vi "Values.vi"(11 "Result Row in":refnum<class "Result Row.lvclass">) -> (2 "Value":refnum<class "Type.lvclass">[](array[class]))   [LabVIEW 2022 SP3, in "Conditum.lvlib" / "Result Row.lvclass"]
uses:
  Result Row.lvclass
  Result Row.lvclass/Result Row.ctl
  Columns/Type/Type.lvclass
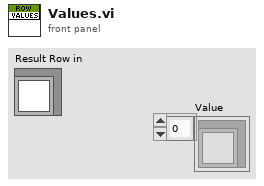
[diagram p1: front panel]
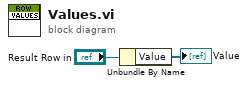
[diagram p0: block diagram]
diagram:
  n1 = Unbundle By Name("Result Row in") -> ("Value"=→"Value":refnum<class "Type.lvclass">[])
